vi "Test Reset Debugger.vi"(8 "error in (no error)":errorcluster, 11 "Test Case In":refnum<class "Debugger Test.lvclass">) -> (0 "error out":errorcluster, 3 "Test Case Out":refnum<class "Debugger Test.lvclass">)   [LabVIEW 2020, in "Debugger Test.lvclass"]
uses:
  Debugger Test.lvclass
  C:/Program Files (x86)/National Instruments/LabVIEW 2020/vi.lib/Astemes/LUnit/Test Case.lvclass
  source/Debugger/Debugger.lvclass
  C:/Users/anton/Documents/GitHub/triarc-debugger/source/Process/Debug Process.lvclass
  source/Debug Data/Raw Debug Data.ctl
  source/Debug Data/Debug Data.lvclass/Debug Data.ctl
  source/Process/Debug Process.lvclass/Debug Process.ctl
  <vilib>/Astemes/LUnit/Test Case.lvclass/Test Case.ctl
  <vilib>/Astemes/LUnit/LUnit Assertion Result.lvclass/LUnit Assertion Result.ctl
  <vilib>/Astemes/LUnit/LUnit Test Case Result.lvclass/LUnit Test Case Result.ctl
  <vilib>/Astemes/LUnit/LUnit Method Result.lvclass/LUnit Method Result.ctl
  01074fa8-ee8a-411d-bc8b-fc92c4f90959.vi
  <vilib>/AdvancedString/Delimited String to 1D String Array.vi
  source/Process/Public/Lifecycle/Get Lifecycle State.vi
  source/Process/Private/SubVIs/Wait for finish.vi
  source/Process/Protected/Messaging/Enqueue Message.vi
  source/Process/Private/SubVIs/Set Lifecycle State.vi
  <vilib>/Astemes/LUnit/Palette/Pass.vi
  <vilib>/Astemes/LUnit/Palette/Fail.vi
  <vilib>/Astemes/LUnit/Compare Variants.vi
  <vilib>/Astemes/LUnit/Describe Comparison.vi
  <vilib>/Astemes/LUnit/Set Assertion Type.vi
  <vilib>/Utility/error.llb/Clear Errors.vi
  <vilib>/Astemes/LUnit/Add test result.vi
  <vilib>/Astemes/LUnit/LUnit Write Passed.vi
  <vilib>/Astemes/LUnit/LUnit Write Message.vi
  <vilib>/Astemes/LUnit/LUnit Write Description.vi
  <vilib>/Astemes/LUnit/Variant to string.vi
  <vilib>/Astemes/LUnit/LUnit Write Assertion Type.vi
  <vilib>/Astemes/LUnit/LUnit Record Assertion Result.vi
  <vilib>/Astemes/LUnit/LUnit Aggregate Assertion Results.vi
  <vilib>/Astemes/LUnit/Assertion Result/LUnit Read Status.vi
  <vilib>/Astemes/LUnit/LUnit Read Message.vi
  <vilib>/Astemes/LUnit/LUnit Read Description.vi
  <vilib>/Astemes/LUnit/Method Result/LUnit Merge Status.vi
  <vilib>/Astemes/LUnit/LUnit Concatenate result strings.vi
  <vilib>/Utility/error.llb/Error Cluster From Error Code.vi
  <vilib>/Utility/Data Type/Get Type Information.vi
  <vilib>/Utility/LVClass/Get LV Class Name.vi
  source/Debug Data/Debug Data.lvclass
  <vilib>/Astemes/LUnit/LUnit Assertion Result.lvclass
  source/Process/Debug Process.lvclass
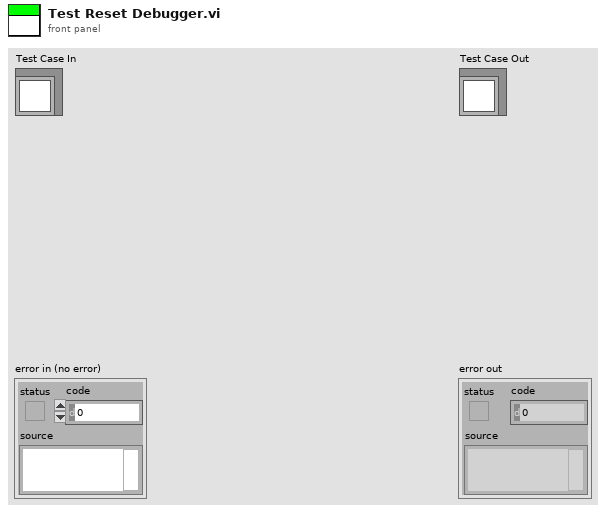
[diagram p1: front panel]
types:
  T1 = typedef "Debug Data.lvclass/Raw Debug Data.ctl" = cluster{"Action":string, "Call Chain":string, "Process":string, "Message":string, "Message Data":variant, "Time":dbl}
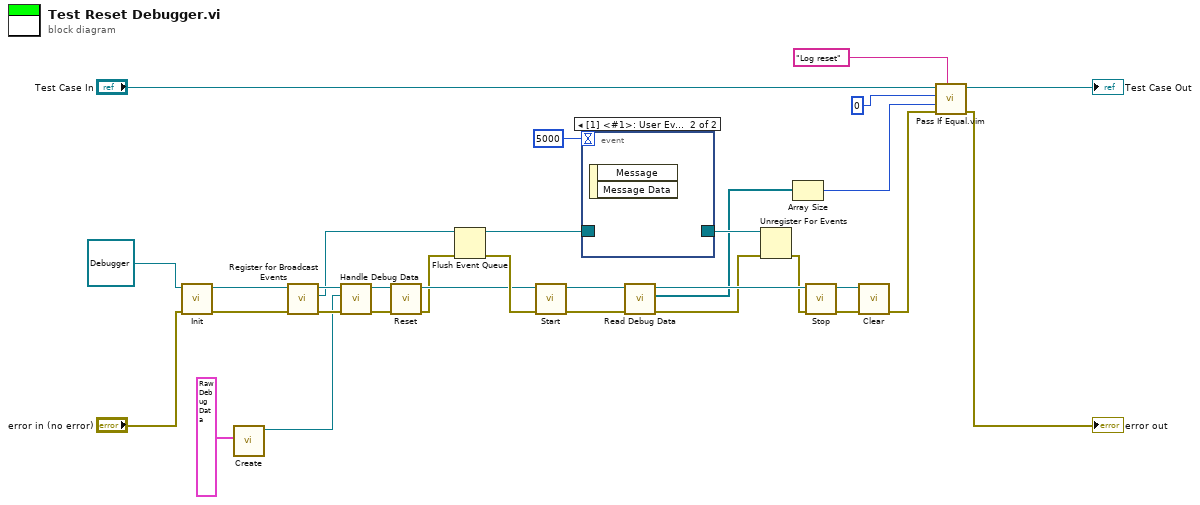
[diagram p0: block diagram]
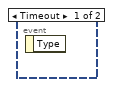
[diagram p2: hidden frame]
diagram:
  n1 = call-dynamic "Init.vi"("error in (no error)"="error in (no error)", "Process In"=refnum<class "Debugger.lvclass"> refnum ("Debug Data Event In 2")) -> ("error out"=w7:errorcluster, "Process Out"=w8:refnum<class "Debugger.lvclass">)  [unwired: 8 in]
  n2 = call "Create.vi"("Debug Data Cluster"=T1 {"Action"="", "Call Chain"="", "Process"="Test", "Message"="", "Message Data"=variant, "Time"=0.0}) -> ("Debug Data out"=w18:refnum<class "Debug Data.lvclass">)  [unwired: 9 in, 1 out]
  n3 = call "Register for Broadcast Events.vi"("error in (no error)"=w7, "Process In"=w8) -> ("error out"=w29:errorcluster, "Event Registration Refnum Out"=w16:refnum<event-registration>, "Process Out"=w25:refnum<class "Debugger.lvclass">)  [unwired: 7 in]
  n4 = call-dynamic "Handle Debug Data.vi"("error in (no error)"=w29, "Debug Data.lvclass"=w18, "Debug Data Event In"=w25) -> ("error out"=w4:errorcluster, "Debug Data Event Out"=w6:refnum<class "Debugger.lvclass">)  [unwired: 7 in]
  n5 = call "Reset.vi"("error in (no error)"=w4, "Debugger in"=w6) -> ("error out"=w3:errorcluster, "Debugger out"=w5:refnum<class "Debugger.lvclass">)  [unwired: 8 in]
  n6 = Flush Event Queue(0:w16, 3:w3) -> (8:w15:refnum<event-registration>, 11:w17:errorcluster)  [unwired: 4 in, 1 out]
  n7 = call "Start.vi"("error in (no error)"=w17, "Process In"=w5) -> ("error out"=w10:errorcluster, "Process Out"=w9:refnum<class "Debugger.lvclass">)  [unwired: 7 in, 1 out]
  n8 = event shown="[1] <#1>: User Event" {
    selector: w15 -> [_ _]
    dyn-events: [_ _] -> w20
    timeout: 5000 -> [_ _]
    event Timeout {
      n9 = event-data() -> ()  [unwired: 1 in, 1 out]
    }
    event User Event {
      n10 = event-data() -> ()  [unwired: 1 in, 2 out]
    }
  }
  n11 = call "Read Debug Data.vi"("error in (no error)"=w10, "Debugger In"=w9) -> ("error out"=w12:errorcluster, "Data Log"=w11:refnum<class "Debug Data.lvclass">[], "Debugger Out"=w28:refnum<class "Debugger.lvclass">)  [unwired: 7 in]
  n12 = Unregister For Events(event registration refnum=w20, error in=w12) -> (error out=w13:errorcluster)
  n13 = Array Size(array=w11) -> (size(s)=w2:i32)
  n14 = call "Stop.vi"("error in (no error)"=w13, "Process In"=w28) -> ("error out"=w26:errorcluster, "Process Out"=w27:refnum<class "Debugger.lvclass">)  [unwired: 7 in, 1 out]
  n15 = call-dynamic "Clear.vi"("error in (no error)"=w26, "Process In"=w27) -> ("error out"=w14:errorcluster)  [unwired: 9 in]
  n16 = call "Pass If Equal.vim"("Description"="Log reset", "error in (no error)"=w14, "Actual"=w2, "Expected"=0 ("size(s)"), "LUnit Test Case In"="Test Case In") -> ("error out"=→"error out":errorcluster, "LUnit Test Case Out"=→"Test Case Out":refnum<class "Debugger Test.lvclass">)  [unwired: 5 in]
